vi "Barcode scanner lisen MIC.vi"(8 "Error out":errorcluster, 10 "port":u16=2000, 11 "service name":string="192.168.1.110") -> (0 "error out 2":errorcluster, 2 "Exit":bool, 3 "data out":string)   [LabVIEW 2015]
uses:
  Galobal variable_TI.vi
  Project Setup/Globle Variable/GR_Servo.vi
panel:
  out "?":bool
  out "Numeric":i32
  out "error out":errorcluster
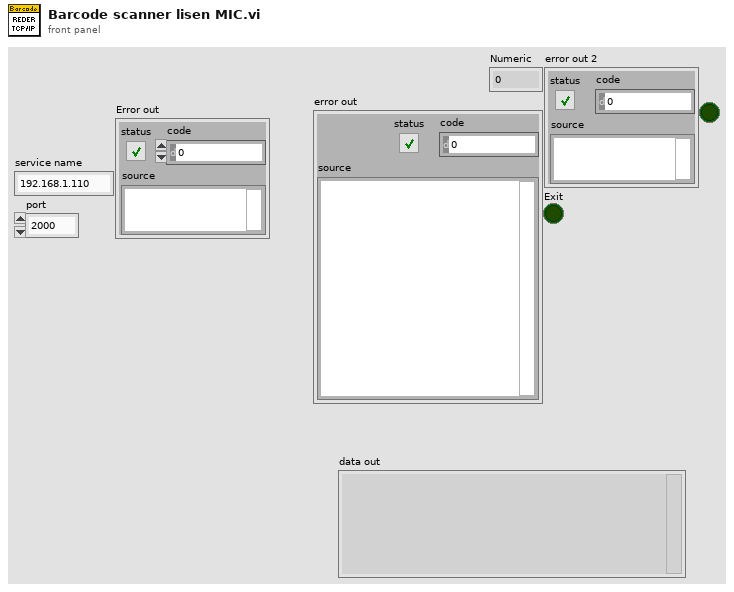
[diagram p1: front panel]
types:
  T1 = cluster{"Load Max(N)":dbl, "Load Min(N)":dbl, "Actuator1 max(mm)":dbl, "Actuator1min(mm)":dbl, "Actuator2 max(mm)":dbl, "Actuator2min(mm)":dbl, "Load Offset":dbl, "Model":string, "MIC Code":string}
  T2 = enum16{"Standard", "Buffered", "CRLF", "Immediate"}
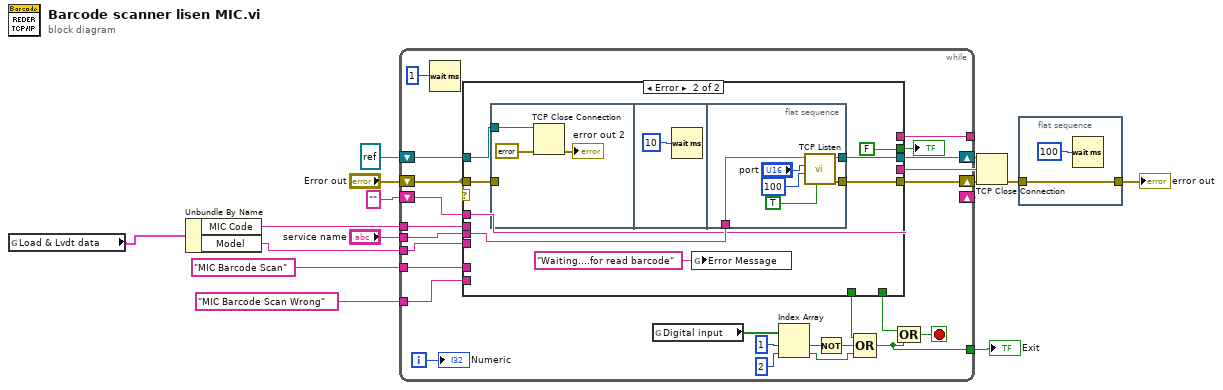
[diagram p0: block diagram]
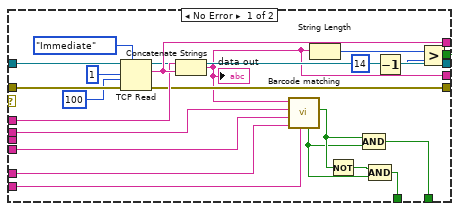
[diagram p2: hidden frame]
diagram:
  n1 = global read "Galobal variable_TI.vi" "Load & Lvdt data"() -> (w1:T1)
  n2 = Unbundle By Name(w1) -> ("MIC Code"=w5:string, "Model"=w4:string)
  n3 = while {
    tunnel: [w37] -> _
    shift-right: [w39] -> w14
    shift-left: refnum<k5> refnum ("connection ID") -> [w36]
    shift-right: [w38] -> w13
    shift-left: "Error out" -> [w35]
    tunnel: "service name" -> [w34]
    shift-right: [w33] -> _
    shift-left: "" -> [w32]
    tunnel: [w22] -> w8
    tunnel: w5 -> [w21]
    tunnel: w4 -> [w20]
    tunnel: "MIC Barcode Scan" ("TFT BARCODE SCANE") -> [w19]
    tunnel: "MIC Barcode Scan Wrong" ("TFT WORNG SCANE") -> [w18]
    i -> [w31]
    stop <- w29 stop-if-true
    n4 = Wait (ms)(milliseconds to wait=u32 1) -> ()  [unwired: 1 out]
    n5 = case shown="Error" w35 {
      tunnel: [w57 w66] -> w39
      tunnel: [w56 w65] -> w38
      tunnel: [w59 _] -> w37
      tunnel: w36 -> [w61 w70]
      tunnel: w35 -> [w60 w69]
      tunnel: w34 -> [_ w68]
      tunnel: [w49 w67] -> w33
      tunnel: w32 -> [w58 w67]
      tunnel: [w53 FALSE] -> w17
      tunnel: w21 -> [w48 _]
      tunnel: w20 -> [w47 _]
      tunnel: w19 -> [w46 _]
      tunnel: w18 -> [w45 _]
      tunnel: [w44 _] -> w16
      tunnel: [w41 _] -> w15
      frame No Error {
        n6 = TCP Read(connection ID=w61, bytes to read=1, error in (no error)=w60, 7:T2."Immediate" ("mode (standard)"), 9:100 ("timeout ms (25000)")) -> (connection ID out=w57:refnum<k5>, data out=w59:string, error out=w56:errorcluster)
        n7 = Concatenate Strings(w58, w59) -> (w49:string)
        "data out" <- w49
        n8 = call "Barcode matching.vi"("TFT WORNG SCANE"=w45, "TFT BARCODE SCANE"=w46, "Model"=w47, "TFT Code"=w48, "Serial data"=w49) -> ("result/trigger"=w43:bool, "Read bit"=w40:bool)  [unwired: 2 in, 3 out]
        n9 = String Length(string=w49) -> (length=w54:i32)
        n10 = Not(x=w43) -> (.not. x?=w42:bool)
        n11 = Compound Arithmetic op=AND(w43, w40) -> (w44:bool)
        n12 = Compound Arithmetic op=AND(w42, w40) -> (w41:bool)
        n13 = Decrement(x=14) -> (x-1=w51:i32)
        n14 = Greater?(x=w54, y=w51) -> (0:w53:bool)
      }
      frame Error {
        n15 = flat-sequence {
          tunnel: w70 -> [w73]
          tunnel: w69 -> [_]
          tunnel: w68 -> [w79]
          tunnel: [w78] -> w66
          tunnel: [w77] -> w65
          frame #0 {
            n16 = TCP Close Connection(connection ID=w73, error in (no error)=errorcluster {"status"=FALSE, "code"=0, "source"=""}) -> (error out=→"error out 2":errorcluster)  [unwired: 1 in, 1 out]
          }
          frame #1 {
            n17 = Wait (ms)(milliseconds to wait=u32 10) -> ()  [unwired: 1 out]
          }
          frame #2 {
            n18 = call <vilib>:"TCP Listen.vi"("resolve remote address (T)"=TRUE, "timeout ms (wait forever: -1)"=100, "port"="port", "service name"=w79) -> ("error out"=w77:errorcluster, "connection ID"=w78:refnum<k5>)  [unwired: 3 in, 3 out]
          }
        }
        n19 = global write "GR_Servo.vi" "Error Message"("Waiting....for read barcode" ("Error Message")) -> ()
      }
    }
    "?" <- w17
    n20 = global read "Galobal variable_TI.vi" "Digital input"() -> (w23:bool[])
    n21 = Index Array(array=w23, index #1=1 ("index"), index #2=2 ("index")) -> (element #1=w26:bool, element #2=w28:bool)
    n22 = Not(x=w26) -> (.not. x?=w27:bool)
    n23 = Compound Arithmetic op=OR(w15, w27, w28) -> (w22:bool)
    n24 = Compound Arithmetic op=OR(w16, w22) -> (w29:bool)
    "Numeric" <- w31
  }
  "Exit" <- w8
  n25 = TCP Close Connection(connection ID=w14, error in (no error)=w13) -> (error out=w7:errorcluster)  [unwired: 1 in, 1 out]
  n26 = flat-sequence {
    tunnel: w7 -> [w82]
    tunnel: [w82] -> w6
    frame #0 {
      n27 = Wait (ms)(milliseconds to wait=u32 100) -> ()  [unwired: 1 out]
    }
  }
  "error out" <- w6
